vi "GetTotalContour.vi"(11 "Refnum in":T2) -> (3 "Segment Information":T1(array[cluster]))   [LabVIEW 2017]
uses:
  <vilib>/vision/Image Controls.llb/IMAQ Image.ctl
panel:
  out "transposed array":dbl[][](array[numeric])
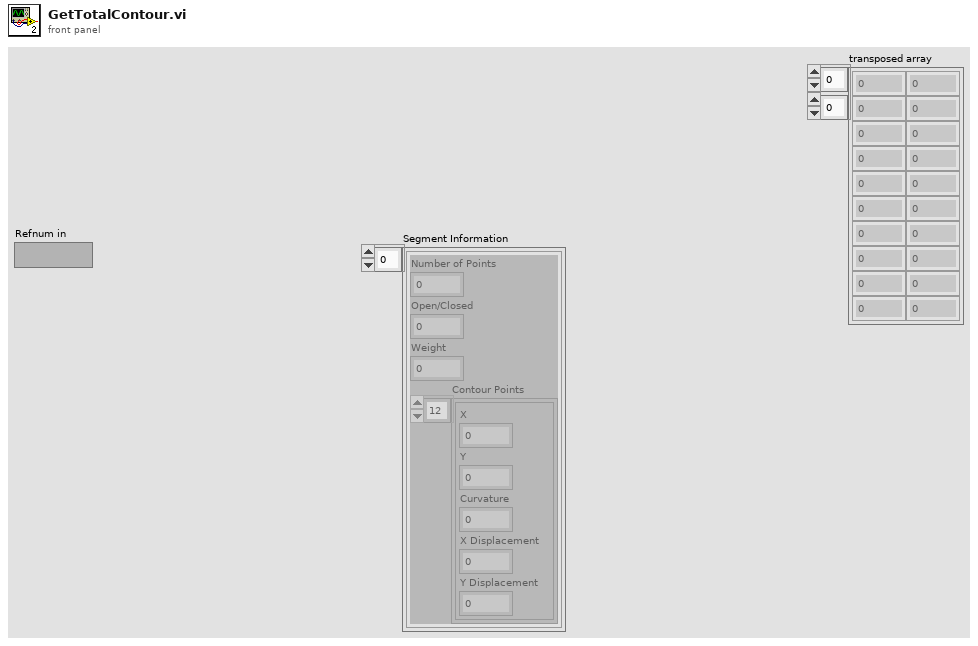
[diagram p1: front panel]
types:
  T1 = cluster{"Number of Points":i32, "Open/Closed":i32, "Weight":dbl, "Contour Points":cluster{"X":dbl, "Y":dbl, "Curvature":dbl, "X Displacement":dbl, "Y Displacement":dbl}[]}[]
  T2 = typedef "IMAQ Image.ctl" = refnum<image>
  T3 = cluster{"Number of Points":i32, "Open/Closed":i32, "Weight":dbl, "Contour Points":cluster{"X":dbl, "Y":dbl, "Curvature":dbl, "X Displacement":dbl, "Y Displacement":dbl}[]}
  T4 = cluster{"X":dbl, "Y":dbl, "Curvature":dbl, "X Displacement":dbl, "Y Displacement":dbl}[]
  T5 = cluster{"X":dbl, "Y":dbl, "Curvature":dbl, "X Displacement":dbl, "Y Displacement":dbl}
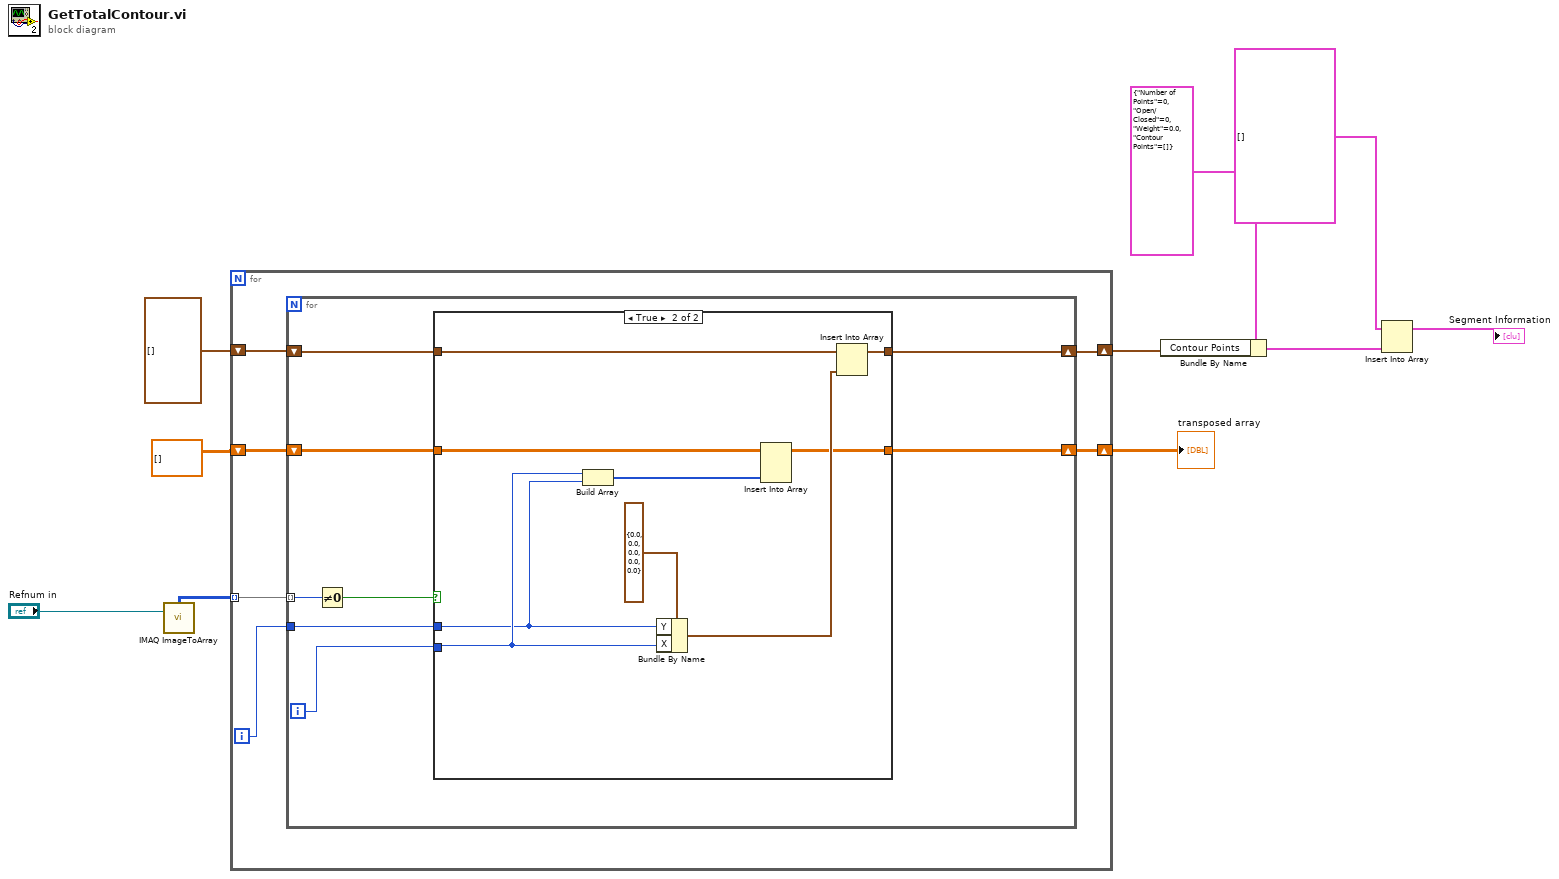
[diagram p0: block diagram]
diagram:
  n1 = call "IMAQ ImageToArray"("Image"="Refnum in") -> ("Image Pixels (U8)"=w4:u8[][])  [unwired: 3 in, 4 out]
  n2 = for {
    shift-right: [w13] -> w1
    shift-left: T4 [] ("Contour Points") -> [w14]
    tunnel: w4 -> [w16] mode=indexing
    shift-right: [w11] -> w2
    shift-left: dbl[][] [] ("transposed array") -> [w12]
    i -> [w15]
    n3 = for {
      tunnel: w16 -> [w24] mode=indexing
      tunnel: w15 -> [w21]
      shift-right: [w19] -> w13
      shift-left: w14 -> [w20]
      shift-right: [w17] -> w11
      shift-left: w12 -> [w18]
      i -> [w22]
      n4 = Not Equal To 0?(x=w24) -> (x != 0?=w23:bool)
      n5 = case shown="True" w23 {
        tunnel: w22 -> [_ w28]
        tunnel: w21 -> [_ w27]
        tunnel: w20 -> [w26 w33]
        tunnel: [w26 w32] -> w19
        tunnel: w18 -> [w25 w30]
        tunnel: [w25 w31] -> w17
        frame False {
        }
        frame True {
          n6 = Build Array(w28, w27) -> (w29:i32[])
          n7 = Bundle By Name(cluster=T5 {"X"=0.0, "Y"=0.0, "Curvature"=0.0, "X Displacement"=0.0, "Y Displacement"=0.0} ("Contour Point"), "Y"=w27, "X"=w28) -> (w34:T5)
          n8 = Insert Into Array(array=w30, new element=w29) -> (w31:dbl[][])  [unwired: 2 in]
          n9 = Insert Into Array(array=w33, new element=w34) -> (w32:T4)  [unwired: 1 in]
        }
      }
    }
  }
  "transposed array" <- w2
  n10 = Bundle By Name(cluster=T3 {"Number of Points"=0, "Open/Closed"=0, "Weight"=0.0, "Contour Points"=[]} ("Contour Information"), "Contour Points"=w1) -> (w7:T3)
  n11 = Insert Into Array(array=T1 [] ("Segment Information"), new element=w7) -> (→"Segment Information":T1)  [unwired: 1 in]
